vi "PID SP LimiterZM.vi"(7 "ZM_State":T2, 8 "REG param":T3={"proportional gain (Kc)"=1.0, "integral time (Ti, s)"=10.0, "derivative time (Td, s)"=1.0, "output high"=100.0, "output high start"=40.0, "output high stop"=40.0, "alr value"=0.0, "output low"=0.0, "output rate (EGU/s)"=5.0, "setpoint max"=100.0, "setpoint rate (EGU/min)"=10.0, "stop rate (EGU/min)"=5.0} {"setpoint max" format="%.2f"; "stop rate (EGU/min)" min=0.001 format="%.2f"; "setpoint rate (EGU/min)" min=0.001 format="%.2f"; "output high stop" format="%.2f"; "output high start" format="%.2f"; "output rate (EGU/s)" min=0.001 format="%.2f"; "output low" format="%.2f"; "alr value" format="%.2f"; "output high" format="%.2f"; "derivative time (Td, s)" format="%.3f"; "integral time (Ti, s)" format="%.3f"; "proportional gain (Kc)" format="%.3f"}, 10 "PV":dbl, 11 "SP":dbl) -> (0 "PID param":T1 {"dt (s)" format="%.3f"; "output rate (EGU/s)" format="%.2f"; "output low" format="%.2f"; "alr value" format="%.2f"; "output high" format="%.2f"; "derivative time (Td, s)" format="%.3f"; "integral time (Ti, s)" format="%.3f"; "proportional gain (Kc)" format="%.3f"}, 1 "End":bool, 2 "T":u32, 3 "output":dbl format="%.2f")   [LabVIEW 2019, in "control.lvlib"]
uses:
  control.lvlib
  Heating/ctl/ZM_State.ctl
  ctl/PID param.ctl
  PID Timing Estimation.vi
  Heating/Heating.lvlib
  Logik/Logik.lvlib
panel:
  # "PID gains"
  # "output param"
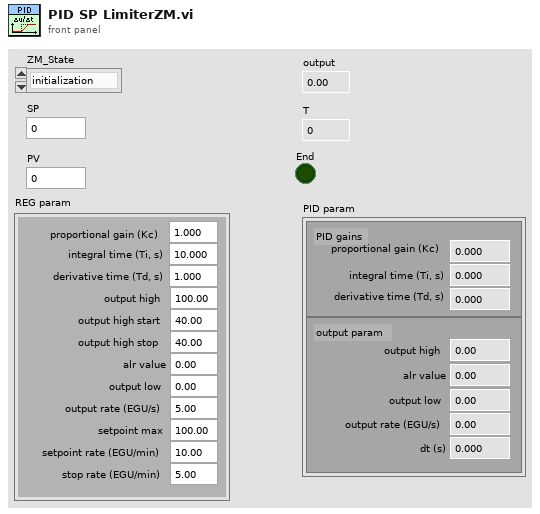
[diagram p1: front panel]
types:
  T1 = typedef "control.lvlib/PID param.ctl" = cluster{"proportional gain (Kc)":dbl, "integral time (Ti, s)":dbl, "derivative time (Td, s)":dbl, "output high":dbl, "alr value":dbl, "output low":dbl, "output rate (EGU/s)":dbl, "dt (s)":dbl}
  T2 = typedef "Heating.lvlib/ZM_State.ctl" = enum8{"initialization", "stop", "start_cmd", "contactor_on_cmd", "heating", "on", "stop_cmd", "power_down", "contactor_off_cmd", "cooling", "restart_delay"}
  T3 = cluster{"proportional gain (Kc)":dbl, "integral time (Ti, s)":dbl, "derivative time (Td, s)":dbl, "output high":dbl, "output high start":dbl, "output high stop":dbl, "alr value":dbl, "output low":dbl, "output rate (EGU/s)":dbl, "setpoint max":dbl, "setpoint rate (EGU/min)":dbl, "stop rate (EGU/min)":dbl}
  T4 = cluster{"proportional gain (Kc)":dbl, "integral time (Ti, s)":dbl, "derivative time (Td, s)":dbl, "output high":dbl, "alr value":dbl, "output low":dbl, "output rate (EGU/s)":dbl, "dt (s)":dbl}
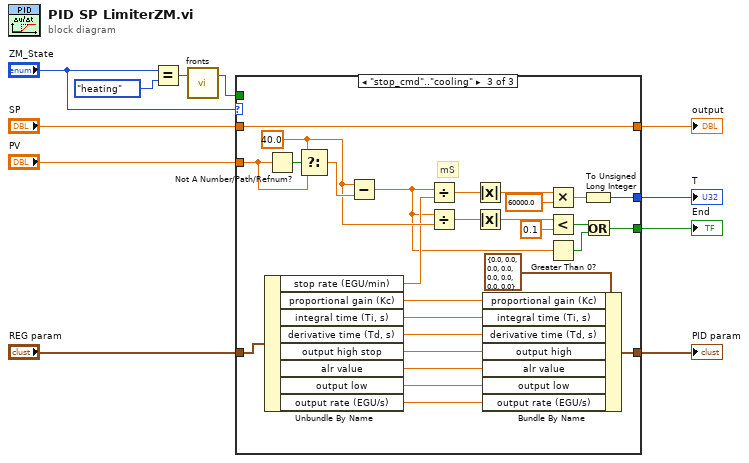
[diagram p0: block diagram]
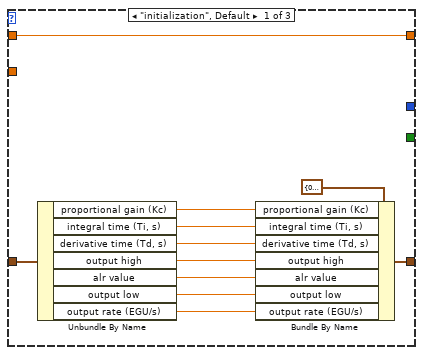
[diagram p2: hidden frame]
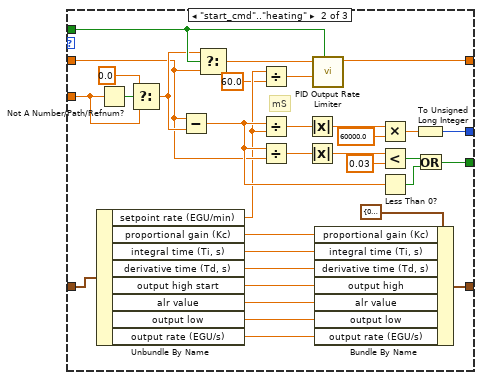
[diagram p3: hidden frame]
diagram:
  n1 = Equal?(x="ZM_State", y=ZM_State."heating" ("ZM_State")) -> (x = y?=w11:bool)
  n2 = call "fronts.vi"("in"=w11) -> ("raise"=w10:bool)  [unwired: 1 in, 1 out]
  n3 = case shown="\"stop_cmd\"..\"cooling\"" "ZM_State" {
    tunnel: "SP" -> [w22 w28 w75]
    tunnel: "PV" -> [_ w52 w82]
    tunnel: [w22 w55 w75] -> w6
    tunnel: [_ w37 w61] -> w5
    tunnel: [_ w33 w58] -> w4
    tunnel: w10 -> [_ w30 _]
    tunnel: "REG param" -> [w14 w47 w66]
    tunnel: [w13 w39 w65] -> w3
    frame "initialization", Default {
      n4 = Unbundle By Name(w14) -> ("proportional gain (Kc)"=w21:dbl, "integral time (Ti, s)"=w20:dbl, "derivative time (Td, s)"=w19:dbl, "output high"=w18:dbl, "alr value"=w17:dbl, "output low"=w16:dbl, "output rate (EGU/s)"=w15:dbl)
      n5 = Bundle By Name(cluster=T4 {"proportional gain (Kc)"=0.0, "integral time (Ti, s)"=0.0, "derivative time (Td, s)"=0.0, "output high"=0.0, "alr value"=0.0, "output low"=0.0, "output rate (EGU/s)"=0.0, "dt (s)"=0.0} ("PID param"), "proportional gain (Kc)"=w21, "integral time (Ti, s)"=w20, "derivative time (Td, s)"=w19, "output high"=w18, "alr value"=w17, "output low"=w16, "output rate (EGU/s)"=w15) -> (w13:T4)
    }
    frame "start_cmd".."heating" {
      # "mS"
      n6 = Unbundle By Name(w47) -> ("setpoint rate (EGU/min)"=w25:dbl, "proportional gain (Kc)"=w46:dbl, "integral time (Ti, s)"=w45:dbl, "derivative time (Td, s)"=w44:dbl, "output high start"=w43:dbl, "alr value"=w42:dbl, "output low"=w41:dbl, "output rate (EGU/s)"=w40:dbl)
      n7 = Not A Number/Path/Refnum?(number/path/refnum=w52) -> (NaN/Path/Refnum?=w53:bool)
      n8 = Select(t=0.0, s=w53, f=w52) -> (s? t:f=w29:dbl)
      n9 = Subtract(x=w28, y=w29) -> (x-y=w34:dbl)
      n10 = Select(t=w29, s=w30, f=w28) -> (s? t:f=w27:dbl)
      n11 = Divide(x=w25, y=60.0 ("x")) -> (x/y=w26:dbl)
      n12 = Divide(x=w34, y=w25) -> (x/y=w50:dbl)
      n13 = Divide(x=w34, y=w28) -> (x/y=w49:dbl)
      n14 = Absolute Value(x=w50) -> (abs(x)=w36:dbl)
      n15 = Absolute Value(x=w49) -> (abs(x)=w48:dbl)
      n16 = call "PID Output Rate Limiter.vi"("reinitialize? (F)"=w30, "output rate (EGU/s)"=w26, "input (controller output)"=w27) -> ("output"=w55:dbl)  [unwired: 7 in, 1 out]
      n17 = Bundle By Name(cluster=T4 {"proportional gain (Kc)"=0.0, "integral time (Ti, s)"=0.0, "derivative time (Td, s)"=0.0, "output high"=0.0, "alr value"=0.0, "output low"=0.0, "output rate (EGU/s)"=0.0, "dt (s)"=0.0} ("PID param"), "proportional gain (Kc)"=w46, "integral time (Ti, s)"=w45, "derivative time (Td, s)"=w44, "output high"=w43, "alr value"=w42, "output low"=w41, "output rate (EGU/s)"=w40) -> (w39:T4)
      n18 = Multiply(x=w36, y=60000.0) -> (x*y=w38:dbl)
      n19 = Less?(x=w48, y=0.03) -> (x < y?=w32:bool)
      n20 = Less Than 0?(x=w34) -> (x < 0?=w31:bool)
      n21 = To Unsigned Long Integer(number=w38) -> (unsigned 32bit integer=w37:u32)
      n22 = Or(x=w32, y=w31) -> (x .or. y?=w33:bool)
    }
    frame "stop_cmd".."cooling" {
      w74 = 40.0 ("t")
      # "mS"
      n23 = Unbundle By Name(w66) -> ("stop rate (EGU/min)"=w64:dbl, "proportional gain (Kc)"=w73:dbl, "integral time (Ti, s)"=w72:dbl, "derivative time (Td, s)"=w71:dbl, "output high stop"=w70:dbl, "alr value"=w69:dbl, "output low"=w68:dbl, "output rate (EGU/s)"=w67:dbl)
      n24 = Not A Number/Path/Refnum?(number/path/refnum=w82) -> (NaN/Path/Refnum?=w83:bool)
      n25 = Select(t=w74, s=w83, f=w82) -> (s? t:f=w81:dbl)
      n26 = Subtract(x=w74, y=w81) -> (x-y=w59:dbl)
      n27 = Divide(x=w59, y=w64) -> (x/y=w79:dbl)
      n28 = Divide(x=w59, y=w74) -> (x/y=w78:dbl)
      n29 = Absolute Value(x=w79) -> (abs(x)=w63:dbl)
      n30 = Absolute Value(x=w78) -> (abs(x)=w77:dbl)
      n31 = Bundle By Name(cluster=T1 {"proportional gain (Kc)"=0.0, "integral time (Ti, s)"=0.0, "derivative time (Td, s)"=0.0, "output high"=0.0, "alr value"=0.0, "output low"=0.0, "output rate (EGU/s)"=0.0, "dt (s)"=0.0} ("PID param"), "proportional gain (Kc)"=w73, "integral time (Ti, s)"=w72, "derivative time (Td, s)"=w71, "output high"=w70, "alr value"=w69, "output low"=w68, "output rate (EGU/s)"=w67) -> (w65:T1)
      n32 = Multiply(x=w63, y=60000.0) -> (x*y=w62:dbl)
      n33 = Less?(x=w77, y=0.1) -> (x < y?=w76:bool)
      n34 = Greater Than 0?(x=w59) -> (x > 0?=w57:bool)
      n35 = To Unsigned Long Integer(number=w62) -> (unsigned 32bit integer=w61:u32)
      n36 = Or(x=w76, y=w57) -> (x .or. y?=w58:bool)
    }
  }
  "output" <- w6
  "PID param" <- w3
  "T" <- w5
  "End" <- w4
